vi "checkStatus.vi"(8 "error in (no error)":errorcluster, 10 "stop":bool, 11 "Pixelfly in":refnum<class "PixelflySA.lvclass">) -> (0 "error out":errorcluster, 2 "stopped?":bool, 3 "Pixelfly out":refnum<class "PixelflySA.lvclass">)   [LabVIEW 2009, in "PixelflySA.lvclass"]
uses:
  PixelflySA.lvclass
  Channels.lvlib
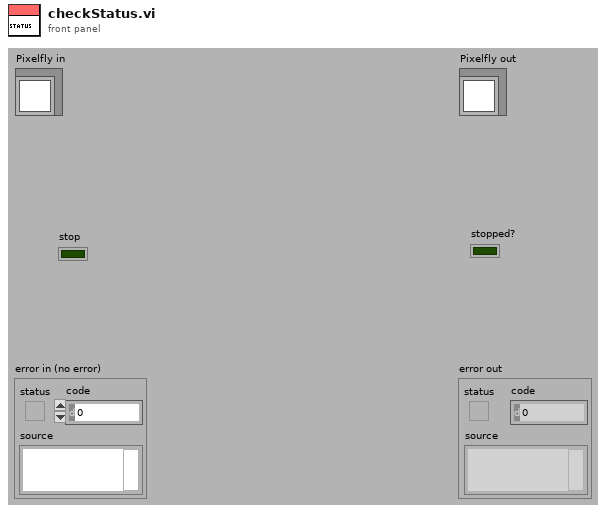
[diagram p1: front panel]
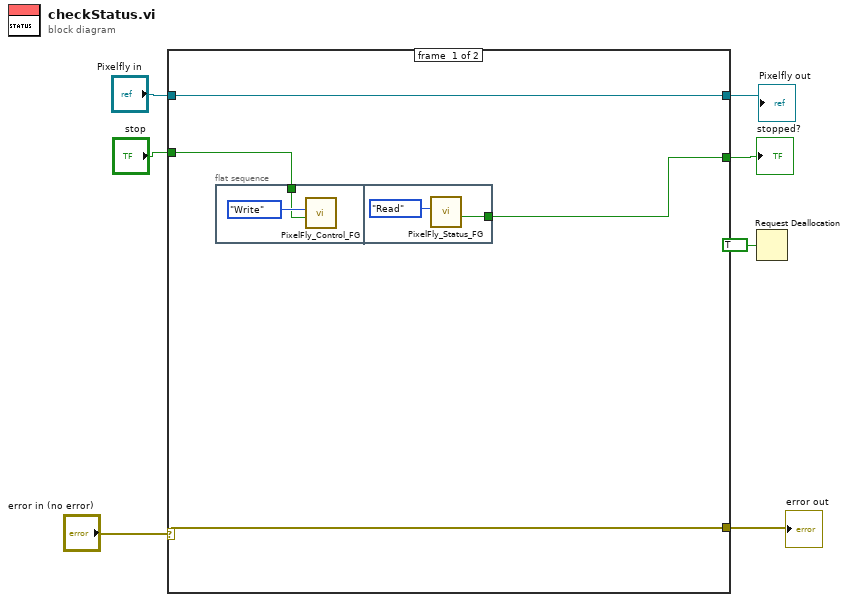
[diagram p0: block diagram]
diagram:
  n1 = case shown="No Error" "error in (no error)" {
    selector: "error in (no error)" -> [w8 w18]
    tunnel: [w8 w18] -> w6
    tunnel: [w11 w17] -> w2
    tunnel: "Pixelfly in" -> [w11 w17]
    tunnel: "stop" -> [w10 w16]
    tunnel: [w9 w16] -> w3
    frame #0 {
      n2 = flat-sequence {
        tunnel: w10 -> [w12]
        tunnel: [w14] -> w9
        frame #0 {
          n3 = call "PixelFly_Control_FG.vi"("stop"=w12, "Action"=enum16{"Write", "Read"}."Write") -> ()  [unwired: 9 in, 1 out]
        }
        frame #1 {
          n4 = call "PixelFly_Status_FG.vi"("Action"=enum16{"Write", "Read"}."Read") -> ("stopped"=w14:bool)  [unwired: 10 in]
        }
      }
    }
    frame #1 {
    }
  }
  "error out" <- w6
  "Pixelfly out" <- w2
  "stopped?" <- w3
  n5 = Request Deallocation(TRUE ("flag")) -> ()
